vi "set_RegArr.vi"(2 "Error Array":errorcluster[](array[cluster]), 3 "Registration Array":T1(array[cluster]), 4 "HGF_SVMonitor":refnum<class "HGF_SVMonitor.lvclass">) -> (1 "HGF_SVMonitor":refnum<class "HGF_SVMonitor.lvclass">)   [LabVIEW 2012, in "HGF_SV.lvlib" / "HGF_SVMonitor.lvclass"]
doc: "update variable cluster. Only those variables will be updated, which did not cause an error."
uses:
  HGF_SVMonitor.lvclass
  HGF_BaseClasses/HGF_NetworkVisitor/HGF_NetworkVisitor.lvclass
  HGF_BaseClasses/HGF_TriggeredEvent/HGF_TriggeredEvent.lvclass
  HGF_SVMonitor.lvclass/HGF_SVMonitor.ctl
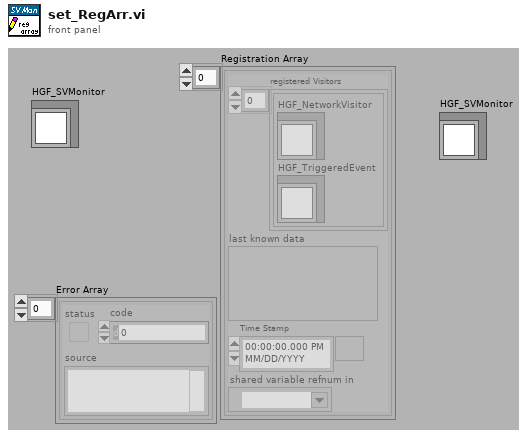
[diagram p1: front panel]
types:
  T1 = cluster{"registered Visitors":cluster{"HGF_NetworkVisitor":refnum<class "HGF_NetworkVisitor.lvclass">, "HGF_TriggeredEvent":refnum<class "HGF_TriggeredEvent.lvclass">}[], "last known data":variant, "Time Stamp":timestamp, "shared variable refnum in":refnum<k21>}[]
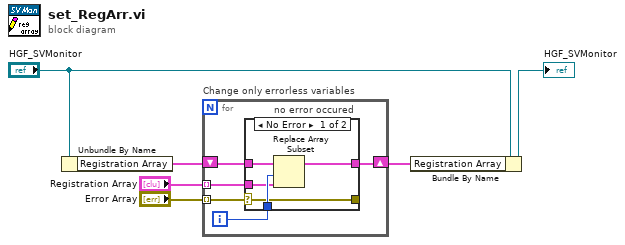
[diagram p0: block diagram]
diagram:
  n1 = Unbundle By Name("HGF_SVMonitor") -> ("Registration Array"=w3:T1)
  n2 = for "Change only errorless variables" {
    tunnel: "Error Array" -> [w11] mode=indexing
    tunnel: "Registration Array" -> [w8] mode=indexing
    shift-right: [w7] -> w2
    shift-left: w3 -> [w10]
    i -> [w9]
    n3 = case "no error occured" shown="No Error" w11 {
      selector: w11 -> [w12 w17]
      tunnel: w10 -> [w16 w18]
      tunnel: w9 -> [w15 _]
      tunnel: w8 -> [w14 _]
      tunnel: [w13 w18] -> w7
      tunnel: [w12 w17] -> _
      frame No Error {
        n4 = Replace Array Subset(array=w16, new element=w14, index=w15) -> (w13:T1)
      }
      frame Error {
      }
    }
  }
  n5 = Bundle By Name(cluster="HGF_SVMonitor", "Registration Array"=w2) -> (→"HGF_SVMonitor":refnum<class "HGF_SVMonitor.lvclass">)
